vi "Time lapse wait for next frame - subvi.vi"(8 "Error In":errorcluster, 10 "Frame Interval (s)":dbl format="%#_13g", 11 "Time of last frame in":u32) -> (0 "Error Out":errorcluster, 1 "Stopped?":bool, 2 "Sec. till next frame":ext(slide), 3 "Time of this frame out (ms)":i32)   [LabVIEW 2014]
uses:
  Shutter Control/Shutter SubVis/control shutters.ctl
  Shutter Control/Shutter SubVis/Global Shutter Variables - SubVI.vi
  TIRF Lock/autofocus-globals.vi
panel:
  in  "stop":bool
  in  "GO NOW!":bool
  in  "Pause":bool
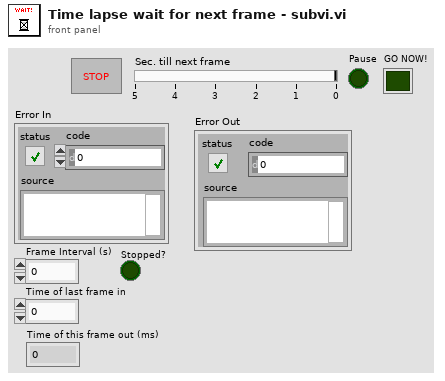
[diagram p1: front panel]
types:
  T1 = typedef "control shutters.ctl" = cluster{"Camera Shutter":bool, "Wheel Speed":u8, "Laser Shutter":enum32{"No Selection", "GFP", "Cy3 Long \nPass", "Cy3", "Cy5", "Off"}}
  T2 = enum32{"No Selection", "GFP", "Cy3 Long \nPass", "Cy3", "Cy5", "Off", "IR"}
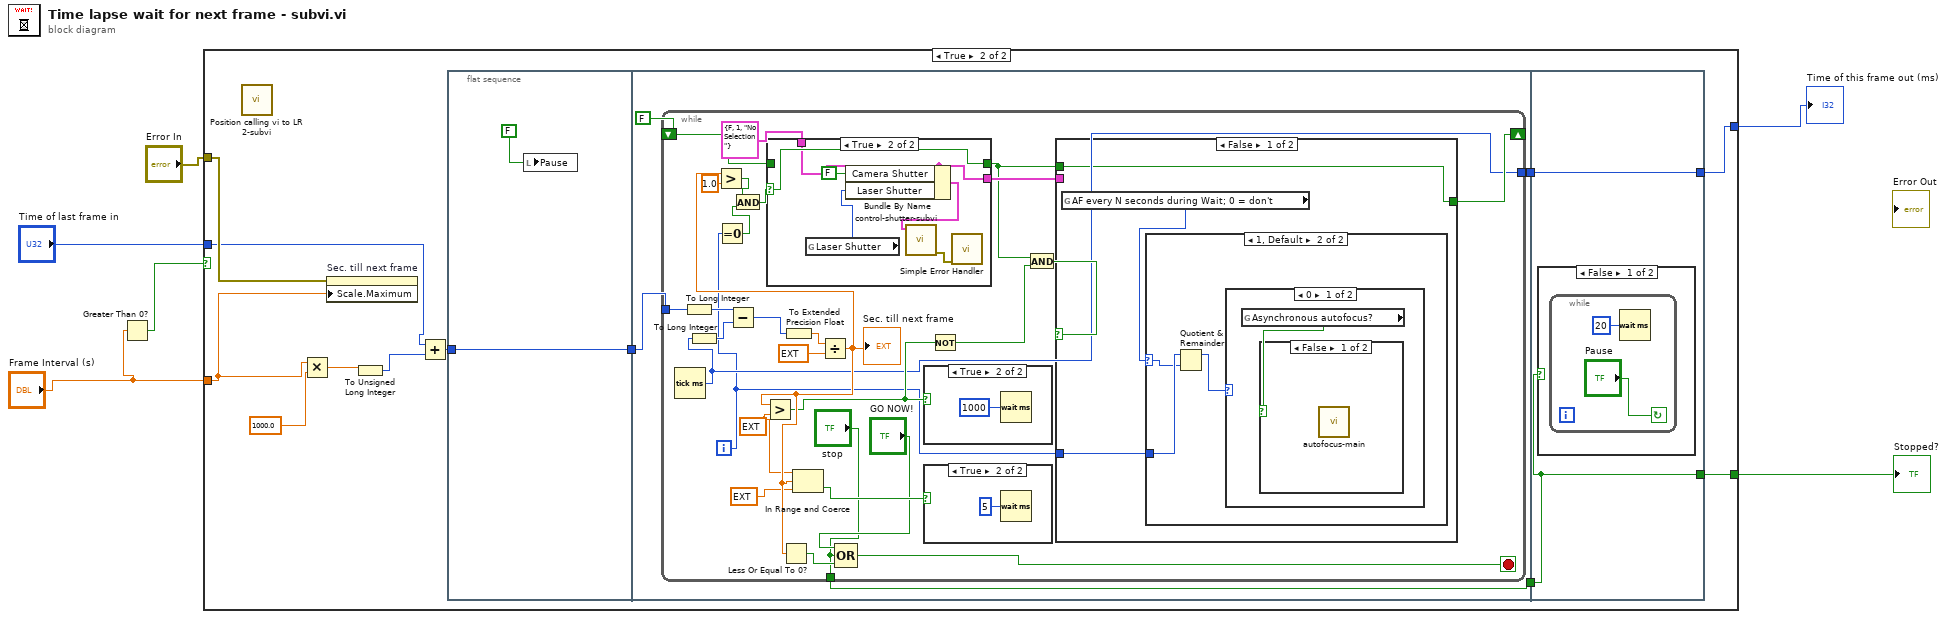
[diagram p0: block diagram]
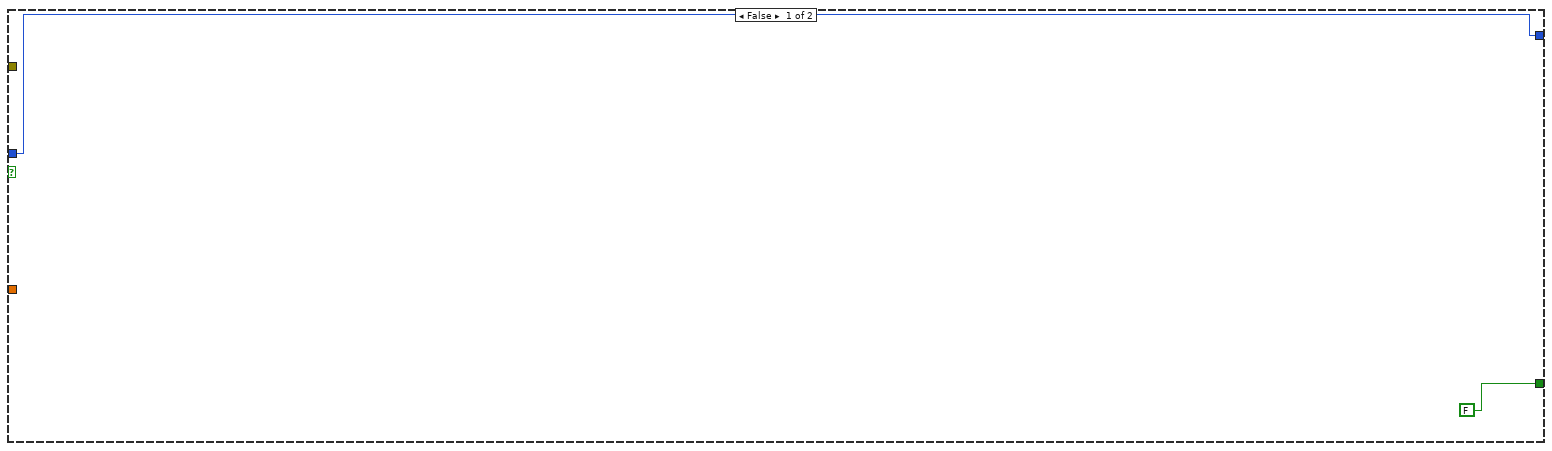
[diagram p2: hidden frame]
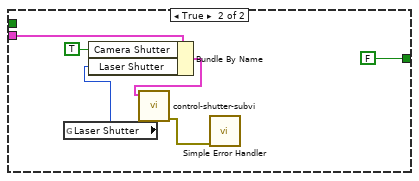
[diagram p6: hidden frame]
diagram:
  n1 = Greater Than 0?(x="Frame Interval (s)") -> (x > 0?=w3:bool)
  n2 = case shown="True" w3 {
    tunnel: "Error In" -> [_ w20]
    tunnel: "Time of last frame in" -> [w8 w15]
    tunnel: "Frame Interval (s)" -> [_ w19]
    tunnel: [w8 w10] -> w2
    tunnel: [FALSE w11] -> w1
    frame False {
    }
    frame True {
      n3 = call "Position calling vi to LR 2-subvi.vi"() -> ()  [unwired: 4 in, 2 out]
      n4 = Multiply(x=w19, y=1000.0) -> (x*y=w17:dbl)
      n5 = property on="Sec. till next frame" class="Slide (strict)"(error in=w20, "Scale.Maximum"=w19) -> ()  [unwired: 1 in, 2 out]
      n6 = To Unsigned Long Integer(number=w17) -> (unsigned 32bit integer=w16:u32)
      n7 = Add(x=w15, y=w16) -> (x+y=w13:u32)
      n8 = flat-sequence {
        tunnel: [w21] -> w14
        tunnel: w13 -> [w21]
        tunnel: w14 -> [w25]
        tunnel: [w24] -> w12
        tunnel: [w23] -> w9
        tunnel: w12 -> [w79]
        tunnel: [w79] -> w11
        tunnel: [w78] -> w10
        tunnel: w9 -> [w78]
        frame #0 {
          n9 = local write "Pause"(FALSE) -> ()
        }
        frame #1 {
          n10 = while {
            shift-right: [w30] -> _
            shift-left: FALSE -> [w54]
            tunnel: w25 -> [w46]
            tunnel: ["stop"] -> w24
            tunnel: [w29] -> w23
            i -> [w28]
            stop <- w38 stop-if-true
            w42 = ext 1.04999999999999999996 ("y")
            n11 = Tick Count (ms)() -> (millisecond timer value=w29:u32)
            n12 = To Long Integer(number=w46) -> (32bit integer=w49:i32)
            n13 = To Long Integer(number=w29) -> (32bit integer=w48:i32)
            n14 = Equal To 0?(x=w28) -> (x = 0?=w51:bool)
            n15 = Subtract(x=w49, y=w48) -> (x-y=w47:i32)
            n16 = To Extended Precision Float(1:w47) -> (0:w45:ext)
            n17 = Divide(x=w45, y=ext 1000.0) -> (x/y=w43:ext)
            "Sec. till next frame" <- w43
            n18 = Greater?(x=w43, y=1.0) -> (0:w52:bool)
            n19 = And(x=w52, y=w51) -> (x .and. y?=w53:bool)
            n20 = Greater?(x=w43, y=w42) -> (0:w34:bool)
            n21 = case shown="True" w53 {
              selector: w53 -> [_ w73]
              tunnel: w54 -> [w71 _]
              tunnel: [w71 w73] -> w27
              tunnel: [w70 w72] -> w32
              tunnel: T1 {"Camera Shutter"=FALSE, "Wheel Speed"=1, "Laser Shutter"=enum."No Selection"} ("Shutter Control") -> [w70 w72]
              frame False {
              }
              frame True {
                n22 = global read "Global Shutter Variables - SubVI.vi" "Laser Shutter"() -> (w75:T2)
                n23 = Bundle By Name(cluster=w72, "Camera Shutter"=FALSE, "Laser Shutter"=w75) -> (w77:T1)
                n24 = call "control-shutter-subvi.vi"("Shutter Control"=w77) -> ("Error Out"=w76:errorcluster)  [unwired: 10 in]
                n25 = call <vilib>:"Simple Error Handler.vi"("error in (no error)"=w76) -> ()  [unwired: 4 in, 5 out]
              }
            }
            n26 = Less Or Equal To 0?(x=w43) -> (x <= 0?=w39:bool)
            n27 = In Range and Coerce(upper limit=w42, x=w43, lower limit=ext 0.01 ("x/y")) -> (In Range?=w40:bool)  [unwired: 1 out]
            n28 = Compound Arithmetic op=OR("GO NOW!", "stop", w39) -> (w38:bool)
            n29 = case shown="True" w34 {
              frame False {
              }
              frame True {
                n30 = Wait (ms)(milliseconds to wait=u32 1000) -> ()  [unwired: 1 out]
              }
            }
            n31 = case shown="True" w40 {
              frame False {
              }
              frame True {
                n32 = Wait (ms)(milliseconds to wait=u32 5) -> ()  [unwired: 1 out]
              }
            }
            n33 = Not(x=w34) -> (.not. x?=w35:bool)
            n34 = And(x=w27, y=w35) -> (x .and. y?=w33:bool)
            n35 = case shown="False" w33 {
              tunnel: w32 -> [_ w67]
              tunnel: [w55 FALSE] -> w30
              tunnel: w28 -> [w56 _]
              tunnel: w27 -> [w55 _]
              frame False {
                n36 = global read "autofocus-globals.vi" "AF every N seconds during Wait; 0 = don't"() -> (w57:u16)
                n37 = case shown="1, Default" w57 {
                  selector: w57 -> [_ w59]
                  tunnel: w56 -> [_ w60]
                  frame 0 {
                  }
                  frame 1, Default {
                    n38 = Quotient & Remainder(x=w60, y=w59) -> (x-y*floor(x/y)=w58:i32)  [unwired: 1 out]
                    n39 = case shown="0" w58 {
                      frame 0 {
                        n40 = global read "autofocus-globals.vi" "Asynchronous autofocus?"() -> (w61:bool)
                        n41 = case shown="False" w61 {
                          frame False {
                            n42 = call "autofocus-main.vi"() -> ()  [unwired: 12 in]
                          }
                          frame True {
                          }
                        }
                      }
                      frame 1, Default {
                      }
                    }
                  }
                }
              }
              frame True {
                n43 = global read "Global Shutter Variables - SubVI.vi" "Laser Shutter"() -> (w65:T2)
                n44 = Bundle By Name(cluster=w67, "Camera Shutter"=TRUE, "Laser Shutter"=w65) -> (w64:T1)
                n45 = call "control-shutter-subvi.vi"("Shutter Control"=w64) -> ("Error Out"=w63:errorcluster)  [unwired: 10 in]
                n46 = call <vilib>:"Simple Error Handler.vi"("error in (no error)"=w63) -> ()  [unwired: 4 in, 5 out]
              }
            }
          }
        }
        frame #2 {
          n47 = case shown="False" w79 {
            frame False {
              n48 = while {
                stop <- "Pause" continue-if-true
                n49 = Wait (ms)(milliseconds to wait=u32 20) -> ()  [unwired: 1 out]
              }
            }
            frame True {
            }
          }
        }
      }
    }
  }
  "Stopped?" <- w1
  "Time of this frame out (ms)" <- w2
